vi "WriteFIFOHeader_HH.vi"(1 "error in":errorcluster, 2 "Destination:":path) -> (0 "error out":errorcluster)   [LabVIEW 2009]
uses:
  FIFOSettings.ctt
  <vilib>/Utility/config.llb/NI_LVConfig.lvlib
panel:
  out "FIFO Settings":T1={"Measurement"={"Binning (ms)"=4719.0, "External Trigger Condition"=14979, "Stop Condition:"=0, "Stop Count"=0.0, "Buffer Size (Photons)"=30000, "No of Channels"=1, "Ext Latch Delay"=0}, "ADC"={"Binning (HH)"=0, "Dither Range"=0, "Count Increment"=0, "Mode"=1}, "SYNC"={"SYNC ZC Level (mV)"=-49.889763, "SYNC Freq Divider"=1, "SYNC Holdoff (ps)"=4.0, "SYNC Threshold (mV)"=-19.607843}, "TAC"={"TAC Range (ns)"=50.0, "TAC Gain"=0, "TAC Offset (%)"=0.0, "TAC Limit Low (%)"=0.0, "TAC Limit High (%)"=100.0}, "Ch 2"={"Ch2 ZC Level (mV)"=-43.137257, "Ch2 Holdoff (ps)"=67.76471, "Ch2 Threshold (mV)"=-49.889763}, "Ch 3"={"Ch3 ZC Level (mV)"=0.0, "Ch3 Holdoff (ps)"=4.0, "Ch3 Threshold (mV)"=200.0}, "Ch 4"={"Ch4 ZC Level (mV)"=0.0, "Ch4 Holdoff (ps)"=4.0, "Ch4 Threshold (mV)"=200.0}, "Ch1"={"Ch1 ZC Level (mV)"=0.0, "Ch1 Holdoff (ps)"=4.0, "Ch1 Threshold (mV)"=200.0}} {"Ch1"."Ch1 Threshold (mV)" min=0 max=1000 format="%.2f"; "Ch1"."Ch1 Holdoff (ps)" min=-99999 max=99999 format="%.2f"; "Ch1"."Ch1 ZC Level (mV)" min=0 max=40 format="%.2f"; "Ch 4"."Ch4 Threshold (mV)" min=0 max=1000 format="%.2f"; "Ch 4"."Ch4 Holdoff (ps)" min=-99999 max=99999 format="%.2f"; "Ch 4"."Ch4 ZC Level (mV)" min=0 max=40 format="%.2f"; "Ch 3"."Ch3 Threshold (mV)" min=0 max=1000 format="%.2f"; "Ch 3"."Ch3 Holdoff (ps)" min=-99999 max=99999 format="%.2f"; "Ch 3"."Ch3 ZC Level (mV)" min=0 max=40 format="%.2f"; "Ch 2"."Ch2 Threshold (mV)" min=-96 max=96 format="%.2f"; "Ch 2"."Ch2 Holdoff (ps)" min=4 max=80 format="%.2f"; "Ch 2"."Ch2 ZC Level (mV)" min=-500 max=80 format="%.2f"; "TAC"."TAC Limit High (%)" min=0 max=100 format="%.2f"; "TAC"."TAC Limit Low (%)" min=5 max=20 format="%.2f"; "TAC"."TAC Offset (%)" min=-96 max=96 format="%.2f"; "TAC"."TAC Gain" min=4 max=80; "TAC"."TAC Range (ns)" min=-500 max=80 format="%.2f"; "SYNC"."SYNC Threshold (mV)" min=5 max=20 format="%.2f"; "SYNC"."SYNC Holdoff (ps)" min=-96 max=96 format="%.2f"; "SYNC"."SYNC Freq Divider" items=["1", "2", "4", "8", "16"]; "SYNC"."SYNC ZC Level (mV)" min=-500 max=80 format="%.2f"; "ADC"."Mode" items=["T3"]; "ADC"."Binning (HH)" items=["1", "2", "4", "8", "16", "32", "64", "128", "256", "512", "1024"]; "ADC"."Count Increment" min=0 max=100; "ADC"."Dither Range" min=1 max=15 step=1; "Measurement"."Ext Latch Delay" min=0 max=255 step=1; "Measurement"."Stop Count" min=-500.0 max=-19.0 format="%.2f"; "Measurement"."Stop Condition:" items=["None", "Photon Count", "Time (s)"]; "Measurement"."External Trigger Condition" min=1 max=16 step=1; "Measurement"."No of Channels" max=14; "Measurement"."Binning (ms)" max=96 format="%.3f"}
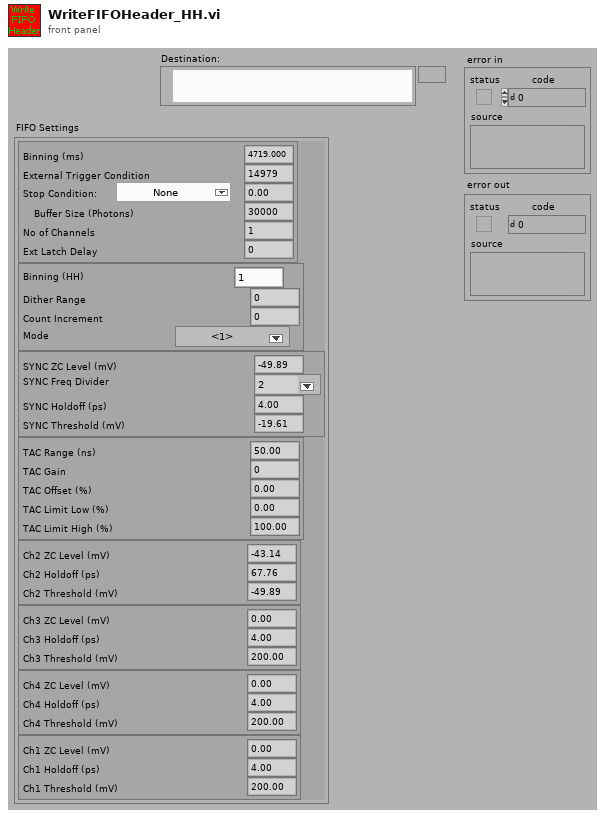
[diagram p1: front panel]
types:
  T1 = typedef "FIFOSettings.ctt" = cluster{"Measurement":cluster{"Binning (ms)":sgl, "External Trigger Condition":u16, "Stop Condition:":u16, "Stop Count":dbl, "Buffer Size (Photons)":u32, "No of Channels":u16, "Ext Latch Delay":i16}, "ADC":cluster{"Binning (HH)":i16, "Dither Range":i16, "Count Increment":i16, "Mode":u16}, "SYNC":cluster{"SYNC ZC Level (mV)":sgl, "SYNC Freq Divider":u16, "SYNC Holdoff (ps)":sgl, "SYNC Threshold (mV)":sgl}, "TAC":cluster{"TAC Range (ns)":sgl, "TAC Gain":i16, "TAC Offset (%)":sgl, "TAC Limit Low (%)":sgl, "TAC Limit High (%)":sgl}, "Ch 2":cluster{"Ch2 ZC Level (mV)":sgl, "Ch2 Holdoff (ps)":sgl, "Ch2 Threshold (mV)":sgl}, "Ch 3":cluster{"Ch3 ZC Level (mV)":sgl, "Ch3 Holdoff (ps)":sgl, "Ch3 Threshold (mV)":sgl}, "Ch 4":cluster{"Ch4 ZC Level (mV)":sgl, "Ch4 Holdoff (ps)":sgl, "Ch4 Threshold (mV)":sgl}, "Ch1":cluster{"Ch1 ZC Level (mV)":sgl, "Ch1 Holdoff (ps)":sgl, "Ch1 Threshold (mV)":sgl}}
  T2 = typedef "NI_LVConfig.lvlib/Config Data RefNum.ctl" = refnum<k1>
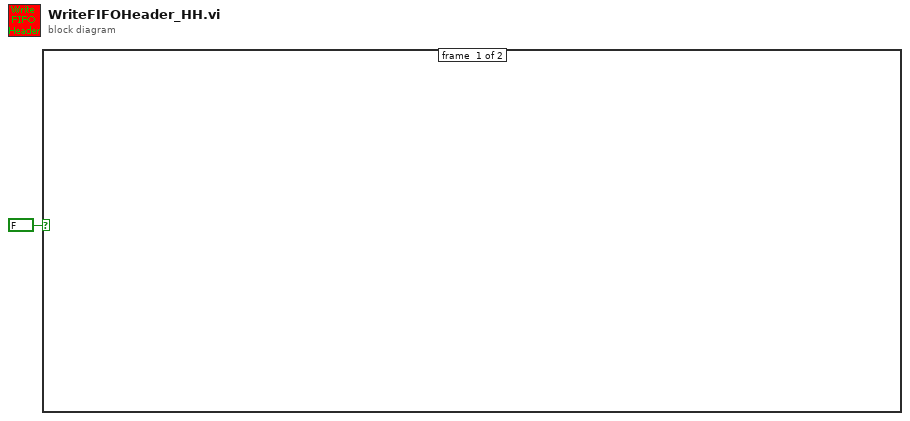
[diagram p0: block diagram]
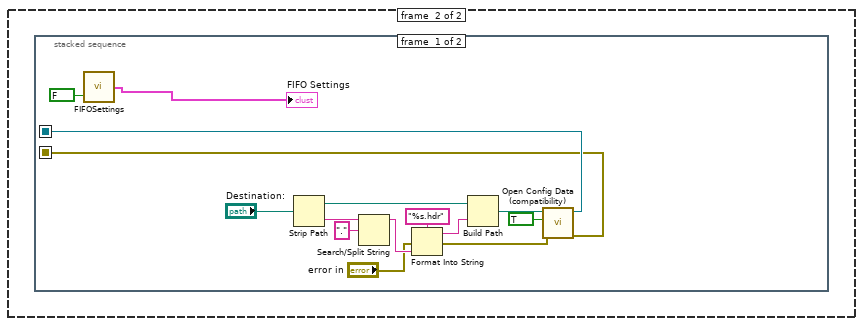
[diagram p2: hidden frame]
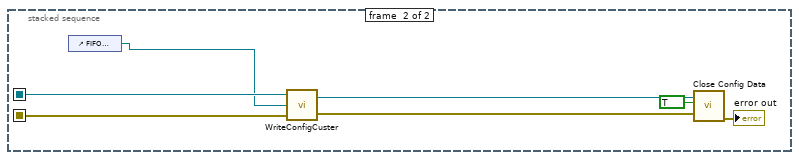
[diagram p3: hidden frame]
diagram:
  n1 = case shown="True" FALSE {
    frame #0 {
    }
    frame #1 {
      n2 = stacked-sequence {
        seq-local: [w6 _] -> [_ w21]
        seq-local: [w5 _] -> [_ w20]
        frame #0 {
          n3 = call "FIFOSettings.vi"("Set/Get"=FALSE) -> ("FIFO Settings(out)"=→"FIFO Settings":T1)  [unwired: 1 in]
          n4 = Strip Path(path="Destination:") -> (stripped path=w12:path, name=w8:string)
          n5 = Search/Split String(string=w8, search string/char (-)=".") -> (substring before match=w11:string)  [unwired: 1 in, 2 out]
          n6 = Format Into String(format string="%s.hdr", error in="error in", w11) -> (resulting string=w13:string, error out=w15:errorcluster)  [unwired: 1 in]
          n7 = Build Path(base path=w12, name or relative path=w13) -> (appended path=w14:path)
          n8 = call <vilib>:"Open Config Data (compatibility).vi"("error in (no error)"=w15, "create file if necessary (T)"=TRUE ("create file if necessary? (T)"), "configuration file path"=w14) -> ("error out"=w5:errorcluster, "refnum"=w6:T2)  [unwired: 6 in, 1 out]
        }
        frame #1 {
          n9 = control-ref of="FIFO Settings"() -> (w17:refnum<vi>)
          n10 = call "WriteConfigCuster.vi"("error in (no error)"=w20, "Ctrl Reference"=w17, "ConfigFile (input)"=w21) -> ("error out"=w18:errorcluster, "ConfigFile (output)"=w19:T2)
          n11 = call "Close Config Data.vi"("error in (no error)"=w18, "write configuration file? (T)"=TRUE ("write configuration file? (F)"), "refnum"=w19) -> ("error out"=→"error out":errorcluster)  [unwired: 8 in]
        }
      }
    }
  }
